vi "Initialize.vi"(8 "error in (no error)":errorcluster, 9 "id query (False)":bool caption="id query (True)", 10 "reset device (False)":bool caption="reset device (True)", 11 "Agilent_3458A in":refnum<class "Agilent_3458A.lvclass">) -> (0 "error out":errorcluster, 3 "Agilent_3458A out":refnum<class "Agilent_3458A.lvclass">)   [LabVIEW 2018, in "DigitizerPlugins.lvlib" / "Agilent_3458A.lvclass"]
uses:
  Agilent_3458A.lvclass
  Y:/Projects/PMUCal/Modules/Digitizer/DigitizerPlugins/DigitizerBaseClass/DigitizerBase.lvclass
  DigitizerBaseClass/DigitizerBase.lvclass/DigitizerBase.ctl
  DigitizerBaseClass/Accessors/Read Handle.vi
  DigitizerBaseClass/Accessors/Write InstRef.vi
  <instrlib>/Agilent 3458/Agilent 3458.lvlib
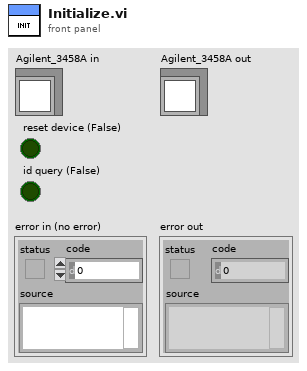
[diagram p1: front panel]
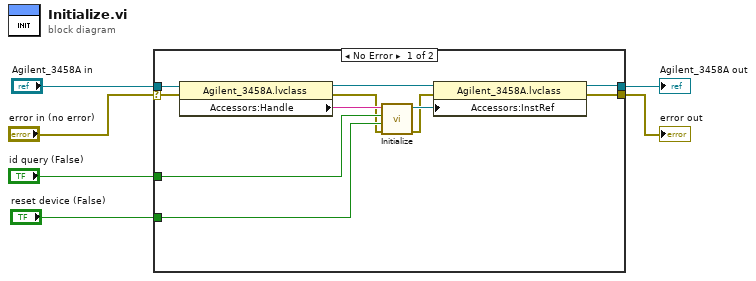
[diagram p0: block diagram]
diagram:
  n1 = case shown="No Error" "error in (no error)" {
    selector: "error in (no error)" -> [w16 w18]
    tunnel: "Agilent_3458A in" -> [w17 w19]
    tunnel: [w8 w19] -> w4
    tunnel: [w7 w18] -> w3
    tunnel: "id query (False)" -> [w13 _]
    tunnel: "reset device (False)" -> [w12 _]
    frame No Error {
      n2 = property class="Agilent_3458A.lvclass"(reference=w17, error in=w16) -> (reference out=w15:refnum<class "Agilent_3458A.lvclass">, error out=w11:errorcluster, "Accessors:Handle"=w14:string)
      n3 = call <instrlib>:"Initialize.vi"("error in (no error)"=w11, "Reset (True)"=w12, "ID Query (True)"=w13, "VISA resource name"=w14) -> ("error out"=w9:errorcluster, "VISA resource name out"=w10:refnum<visa-resource-name>)  [unwired: 6 in]
      n4 = property class="Agilent_3458A.lvclass"(reference=w15, error in=w9, "Accessors:InstRef"=w10) -> (reference out=w8:refnum<class "Agilent_3458A.lvclass">, error out=w7:errorcluster)
    }
    frame Error {
    }
  }
  "error out" <- w3
  "Agilent_3458A out" <- w4
